vi "ExCircularBufferExample.vi"() -> ()   [LabVIEW 2010]
panel:
  in  "Trigger Edge":u32(ring)=1 items=["", "Positive (leading) edge", "Negative (falling) Edge"]
  in  "Trigger/Timing Mode":u32(ring)=1 items=["N/A", "FreeRun/Timed", "Single Trigger (PM only)", "Ext Sync/Strobed", "Bulb (PM only)", "Variable (PM only)", "Flash Mode (PM only)"]
  in  "Temperature":dbl=-10.0 format="%.2f"
  in  "Exposure":dbl min=0.0 step=0.001 format="%.3f"
  in  "stop":bool
  in  "Store":bool
  out "error out":errorcluster
  in  "error in (no error)":errorcluster
  # "ExCircularBufferExample:\nThis example collects a full image using circular buffers.\nNote: not all cameras support circular buffers."
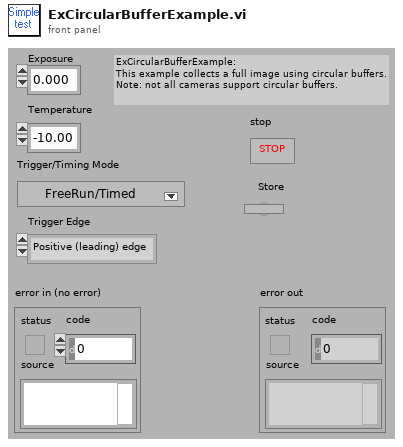
[diagram p1: front panel]
types:
  T1 = cluster{"acquire Mode\nSync-Focus \nNote: not all \ncameras support \nthis mode":i32, "Exposure":dbl, "Number of frames":i32, "Software Accumulations":i32}
  T2 = cluster{"Camera Handle":u32, "Pulser Handle":u32, "File Handle":u32, "Display Handle":u32, "Image Handle":u32}
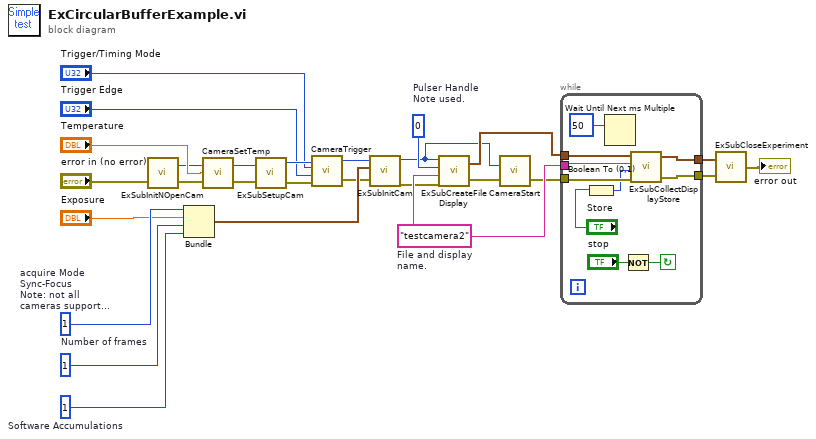
[diagram p0: block diagram]
diagram:
  w19 = 0  # Pulser Handle Note used.
  w25 = 1  # Number of frames
  w26 = 1  # acquire Mode Sync-Focus  Note: not all  cameras support  this mode
  w24 = 1  # Software Accumulations
  w27 = "testcamera2"  # File and display  name.
  n1 = call "ExSubInitNOpenCam.vi"("error in (no error)"="error in (no error)") -> ("Camera Handle"=w5:u32, "error out"=w6:errorcluster)
  n2 = Bundle("acquire Mode\nSync-Focus \nNote: not all \ncameras support \nthis mode"=w26, "Exposure"="Exposure", "Number of frames"=w25, "Software Accumulations"=w24) -> (w21:T1)  [unwired: 1 in]
  n3 = call <userlib>:"CameraSetTemp.vi"("error in (no error)"=w6, "Temperature"="Temperature", "Camera Handle"=w5) -> ("error out"=w4:errorcluster, "Camera Handle"=w3:u32)
  n4 = call "ExSubSetupCam.vi"("error in (no error)"=w4, "Camera Handle"=w3) -> ("error out"=w10:errorcluster, "Camera Handle"=w12:u32)
  n5 = call <userlib>:"CameraTrigger.vi"("error in"=w10, "Trigger Edge"="Trigger Edge", "Timing Mode"="Trigger/Timing Mode", "Camera Handle"=w12) -> ("error out"=w13:errorcluster, "Camera Handle"=w11:u32)
  n6 = call "ExSubInitCam.vi"("error in (no error)"=w13, "Camera Information"=w21, "Camera Handle"=w11) -> ("error out"=w20:errorcluster, "Camera Handle"=w17:u32)
  n7 = call "ExSubCreateFileDisplay.vi"("error in (no error)"=w20, "File and Display Name"=w27, "Pulser Handle"=w19, "Camera Handle"=w17) -> ("error out"=w8:errorcluster, "Handles Out"=w18:T2)
  n8 = call <userlib>:"CameraStart.vi"("error in"=w8, "Camera Handle"=w17) -> ("error out"=w9:errorcluster)  [unwired: 1 out]
  n9 = while {
    tunnel: w18 -> [w36]
    tunnel: w9 -> [w34]
    tunnel: w27 -> [w35]
    tunnel: [w32] -> w15
    tunnel: [w33] -> w16
    stop <- w30 continue-if-true
    n10 = Boolean To (0,1)(Boolean="Store") -> (0, 1=w28:i16)
    n11 = Wait Until Next ms Multiple(millisecond multiple=50) -> ()  [unwired: 1 out]
    n12 = Not(x="stop") -> (.not. x?=w30:bool)
    n13 = call "ExSubCollectDisplayStore.vi"("error in (no error)"=w34, "Store flag"=w28, "Display Title"=w35, "Handle Cluster"=w36) -> ("error out"=w32:errorcluster, "Handle Cluster Out"=w33:T2)  [unwired: 1 out]
  }
  n14 = call "ExSubCloseExperiment.vi"("error in (no error)"=w15, "Handles In"=w16) -> ("error out"=→"error out":errorcluster)
